vi "RunFullWormRailsTwoColors.vi"() -> ()   [LabVIEW 2019]
uses:
  Parameters.ctl
  FullWormRailsTwoColors/FullWormRailsTwoColorsInputCluster.ctl
  FullWormRailsTwoColors.lvclass
  D:/Github_repos/ProjectAPI/LabviewVIs/StimulusObject.lvclass
panel:
  in  "FullWormRailsTwoColorsInputCluster":T1={"Constant Intensity (uW/mm^2, negative is blue)"=0.0, "dot radius (mm)"=0.3, "BlueIntensity (uW/mm^2, negative is blue)"=[], "Durations (s)"=[], "Inter trigger interval (s)"=10.0, "RedIntensity (uW/mm^2, positive is red)"=[]}
  out "error IO":errorcluster
  in  "SSH password 2":string
  in  "SSH user name 2":string
  in  "Start":bool
  in  "Wait Before Recording (s)":u32
  in  "SSH password":string
  in  "username@della.princeton.edu":string
  in  "Last Experiment of the Day":bool
  in  "Tags":string
  out "Parameters":T2 {"FW_WormLengthSD" format="%#.6e"}
  # "Faux Worm Drawing"
  # "Tracking"
  # "Temporal Calibration"
  # "Stimulus Generation"
  # "Median Filtering"
  # "Experimental Settings"
  # "Camera and Projector Settings"
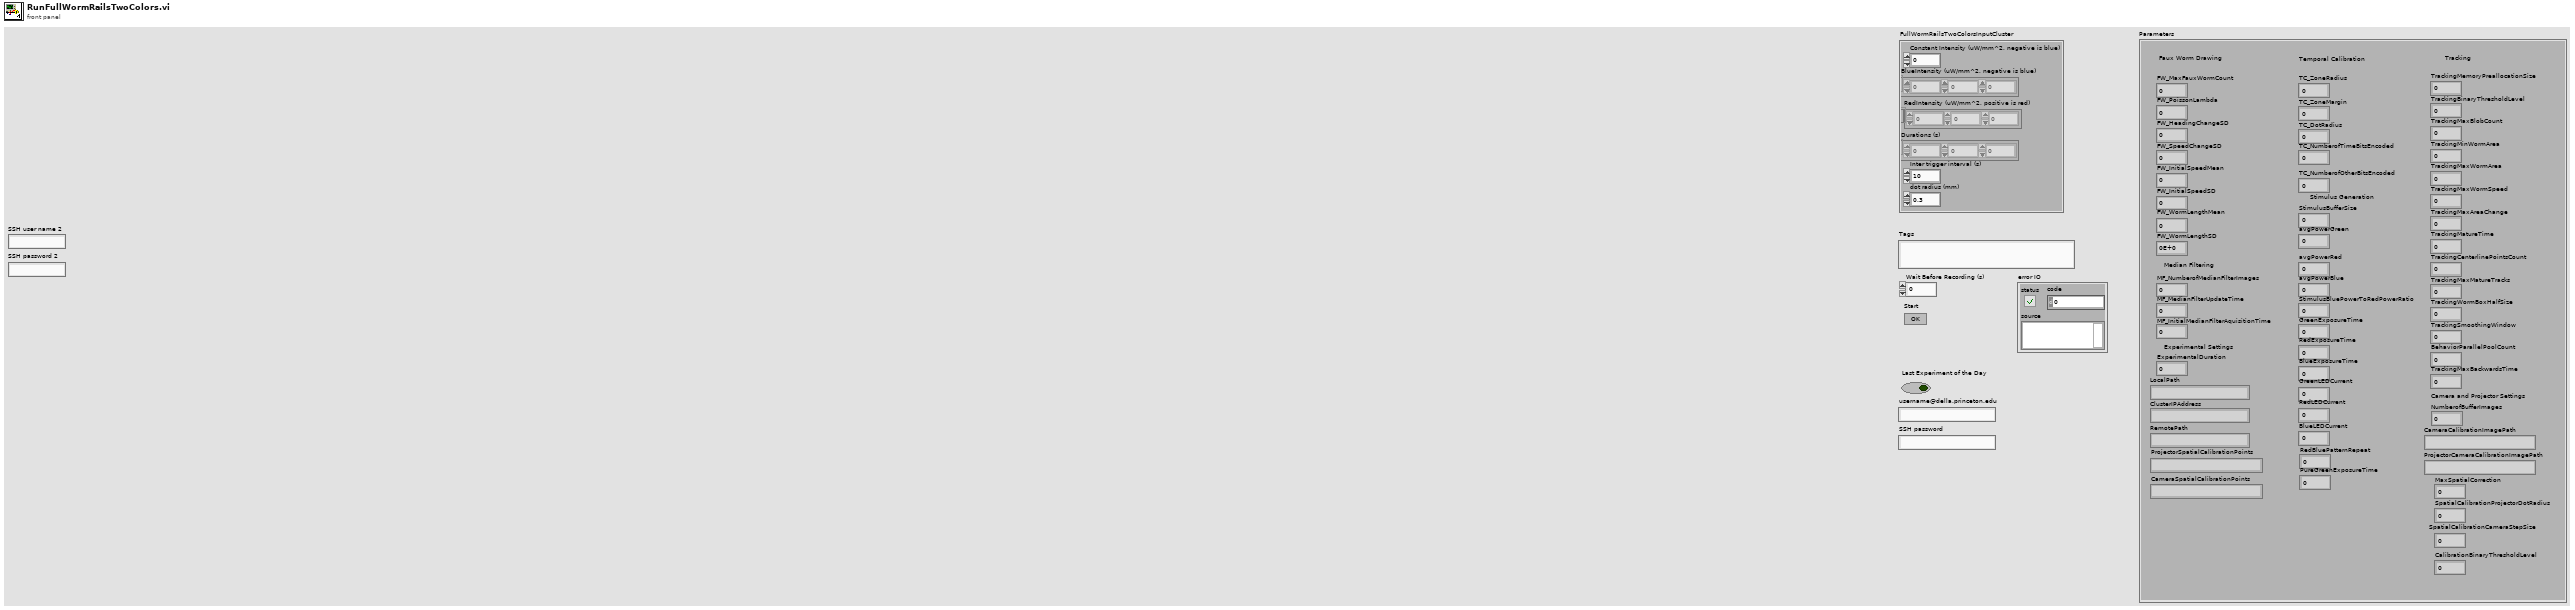
[diagram p1: front panel]
types:
  T1 = typedef "FullWormRailsTwoColors.lvclass/FullWormRailsTwoColorsInputCluster.ctl" = cluster{"Constant Intensity (uW/mm^2, negative is blue)":sgl, "dot radius (mm)":sgl, "BlueIntensity (uW/mm^2, negative is blue)":sgl[], "Durations (s)":sgl[], "Inter trigger interval (s)":dbl, "RedIntensity (uW/mm^2, positive is red)":sgl[]}
  T2 = typedef "Parameters.ctl" = cluster{"FW_MaxFauxWormCount":i32, "FW_PoissonLambda":dbl, "FW_HeadingChangeSD":dbl, "FW_SpeedChangeSD":dbl, "FW_InitialSpeedMean":dbl, "FW_InitialSpeedSD":dbl, "FW_WormLengthMean":dbl, "FW_WormLengthSD":dbl, "MF_NumberofMedianFilterImages":i32, "MF_MedianFilterUpdateTime":i32, "MF_InitialMedianFilterAquisitionTime":dbl, "ExperimentalDuration":i32, "TC_ZoneRadius":i32, "TC_ZoneMargin":i32, "TC_DotRadius":dbl, "TC_NumberofTimeBitsEncoded":i32, "TC_NumberofOtherBitsEncoded":i32, "NumberofBufferImages":sgl, "CameraCalibrationImagePath":string, "ProjectorCameraCalibrationImagePath":string, "StimulusBufferSize":i32, "TrackingMemoryPreallocationSize":i32, "TrackingBinaryThresholdLevel":sgl, "TrackingMaxBlobCount":i32, "TrackingMinWormArea":dbl, "TrackingMaxWormArea":dbl, "TrackingMaxWormSpeed":dbl, "TrackingMaxAreaChange":dbl, "TrackingMatureTime":i32, "TrackingCenterlinePointsCount":i32, "TrackingMaxMatureTracks":i32, "TrackingWormBoxHalfSize":i32, "TrackingSmoothingWindow":i32, "BehaviorParallelPoolCount":i32, "LocalPath":string, "GreenExposureTime":i32, "RedExposureTime":i32, "BlueExposureTime":i32, "ClusterIPAddress":string, "RemotePath":string, "GreenLEDCurrent":u8, "RedLEDCurrent":u8, "BlueLEDCurrent":u8, "avgPowerGreen":sgl, "avgPowerRed":sgl, "avgPowerBlue":sgl, "StimulusBluePowerToRedPowerRatio":sgl, "TrackingMaxBackwardsTime":i32, "MaxSpatialCorrection":dbl, "ProjectorSpatialCalibrationPoints":string, "SpatialCalibrationProjectorDotRadius":i32, "SpatialCalibrationCameraStepSize":dbl, "CameraSpatialCalibrationPoints":string, "CalibrationBinaryThresholdLevel":dbl, "RedBluePatternRepeat":i32, "PureGreenExposureTime":i32}
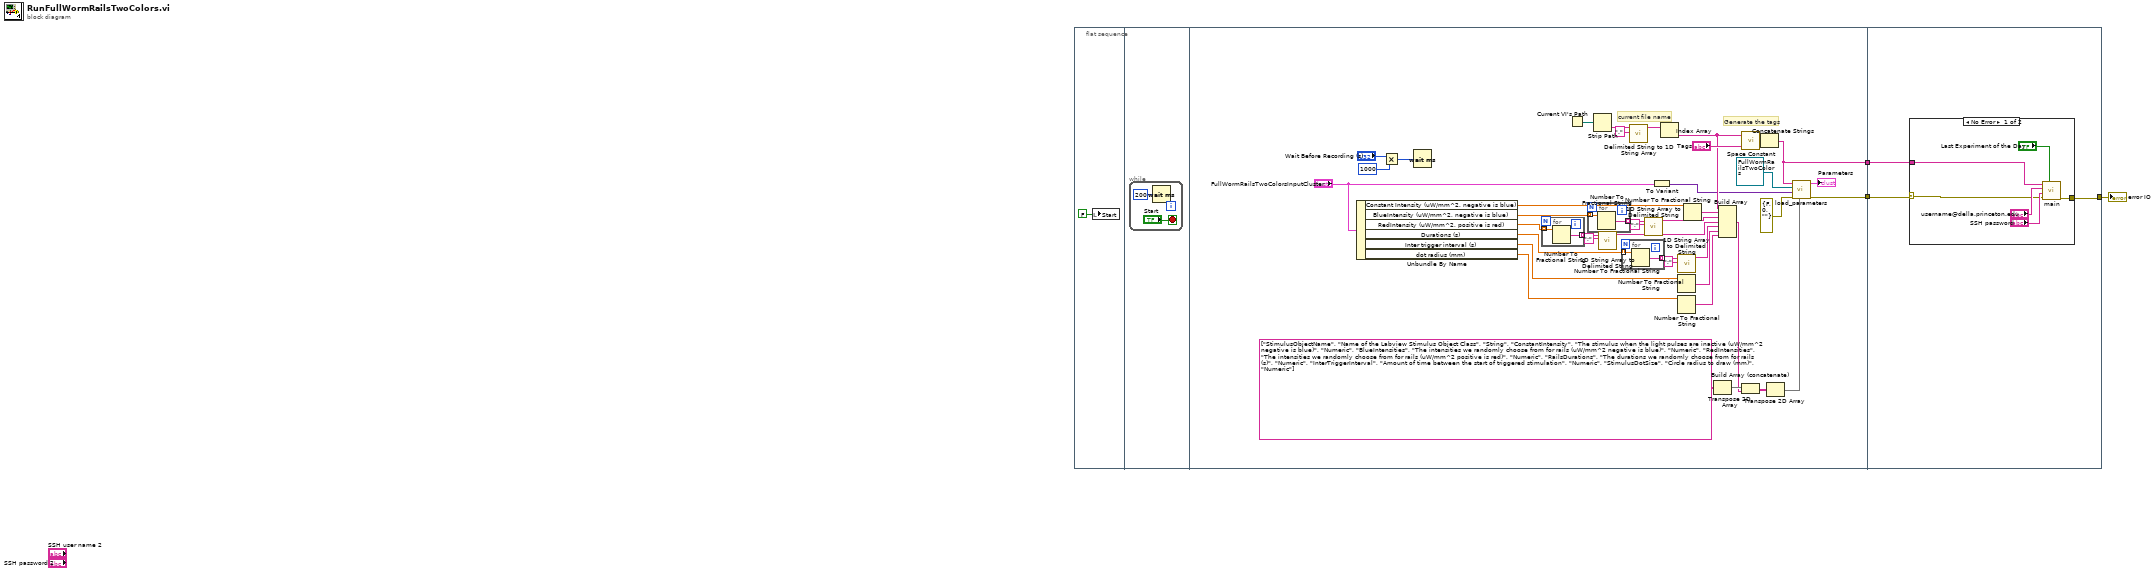
[diagram p0: block diagram]
diagram:
  n1 = flat-sequence {
    tunnel: [w46] -> w3
    tunnel: [w36] -> w2
    tunnel: w2 -> [w54]
    tunnel: w3 -> [w55]
    tunnel: [w53] -> w1
    frame #0 {
      n2 = local write "Start"(FALSE ("Start")) -> ()
    }
    frame #1 {
      n3 = while {
        stop <- "Start" stop-if-true
        n4 = Wait (ms)(milliseconds to wait=u32 200) -> ()  [unwired: 1 out]
      }
    }
    frame #2 {
      # "current file name"
      # "Generate the tags"
      n5 = Unbundle By Name("FullWormRailsTwoColorsInputCluster") -> ("Constant Intensity (uW/mm^2, negative is blue)"=w25:sgl, "BlueIntensity (uW/mm^2, negative is blue)"=w24:sgl[], "RedIntensity (uW/mm^2, positive is red)"=w18:sgl[], "Durations (s)"=w10:sgl[], "Inter trigger interval (s)"=w16:dbl, "dot radius (mm)"=w14:sgl)
      n6 = Multiply(x="Wait Before Recording (s)", y=u32 1000) -> (x*y=w33:u32)
      n7 = Wait (ms)(milliseconds to wait=w33) -> ()  [unwired: 1 out]
      n8 = for {
        tunnel: w18 -> [w50] mode=indexing
        tunnel: [w49] -> w20 mode=indexing
        n9 = Number To Fractional String(number=w50) -> (F-format string=w49:string)  [unwired: 3 in]
      }
      n10 = Current VI's Path() -> (path=w31:path)
      n11 = for {
        tunnel: w24 -> [w52] mode=indexing
        tunnel: [w51] -> w23 mode=indexing
        n12 = Number To Fractional String(number=w52) -> (F-format string=w51:string)  [unwired: 3 in]
      }
      n13 = Strip Path(path=w31) -> (name=w30:string)  [unwired: 1 out]
      n14 = call <vilib>:"1D String Array to Delimited String.vi"("delimiter"=";", "string array"=w20) -> ("delimited string"=w17:string)  [unwired: 9 in]
      n15 = for {
        tunnel: w10 -> [w48] mode=indexing
        tunnel: [w47] -> w12 mode=indexing
        n16 = Number To Fractional String(number=w48) -> (F-format string=w47:string)  [unwired: 3 in]
      }
      n17 = call <vilib>:"Delimited String to 1D String Array.vi"("delimiter"=".", "delimited string"=w30) -> ("string array"=w28:string[])  [unwired: 9 in]
      n18 = call <vilib>:"1D String Array to Delimited String.vi"("delimiter"=";", "string array"=w23) -> ("delimited string"=w21:string)  [unwired: 9 in]
      n19 = To Variant(anything="FullWormRailsTwoColorsInputCluster") -> (Variant=w26:variant)
      n20 = Index Array(array=w28) -> (element=w27:string)  [unwired: 1 in]
      n21 = call <vilib>:"1D String Array to Delimited String.vi"("delimiter"=";", "string array"=w12) -> ("delimited string"=w9:string)  [unwired: 9 in]
      n22 = Number To Fractional String(number=w16) -> (F-format string=w15:string)  [unwired: 3 in]
      n23 = Number To Fractional String(number=w14) -> (F-format string=w13:string)  [unwired: 3 in]
      n24 = Number To Fractional String(number=w25) -> (F-format string=w44:string)  [unwired: 3 in]
      n25 = Transpose 2D Array(2D array=string[][] [["StimulusObjectName", "Name of the Labview Stimulus Object Class", "String"], ["ConstantIntensity", "The stimulus when the light pulses are inactive (uW/mm^2 negative is blue)", "Numeric"], ["BlueIntensities", "The intensities we randomly choose from for rails (uW/mm^2 negative is blue)", "Numeric"], ["RedIntensities", "The intensities we randomly choose from for rails (uW/mm^2 positive is red)", "Numeric"], ["RailsDurations", "The durations we randomly choose from for rails (s)", "Numeric"], ["InterTriggerInterval", "Amount of time between the start of triggered stimulation", "Numeric"], ["StimulusDotSize", "Circle radius to draw (mm)", "Numeric"]]) -> (transposed array=w42:string[][])
      n26 = Build Array(w27, w44, w21, w17, w9, w15, w13) -> (w41:string[])
      n27 = Build Array (concatenate)(w42, w41) -> (w40:string[][])
      n28 = call <vilib>:"Space Constant.vi"() -> ("String"=w38:string)
      n29 = Concatenate Strings(w27, w38, "Tags") -> (w36:string)
      n30 = Transpose 2D Array(2D array=w40) -> (transposed array=w37:string[][])
      n31 = call "load_parameters.vi"("additional loaded parameters to write"=w37, "error in (no error)"=errorcluster {"status"=FALSE, "code"=0, "source"=""}, "StimulusObject Parameters"=w26, "StimulusObjectClassInput"=refnum<class "FullWormRailsTwoColors.lvclass"> refnum ("FullWormRailsTwoColors.lvclass"), "Tags"=w36) -> ("error out"=w46:errorcluster, "Parameters"=→"Parameters":T2)  [unwired: 4 in, 1 out]
    }
    frame #3 {
      n32 = case shown="No Error" w55 {
        selector: w55 -> [w58 w62]
        tunnel: [w57 w62] -> w53
        tunnel: w54 -> [w56 _]
        frame No Error {
          n33 = call "main.vi"("Last Experiment of the Day"="Last Experiment of the Day", "error in"=w58, "SSH password"="SSH password", "SSH user name"="username@della.princeton.edu", "Tags"=w56) -> ("error out"=w57:errorcluster)  [unwired: 6 in]
        }
        frame Error {
        }
      }
    }
  }
  "error IO" <- w1
